vi "GEOM_findAmplifierbyCoord.vi"(9 "amplifiers":T1[](array[typedef]) {"fliped" items=["none", "horizontal", "vertical"]; "type" items=["LL", "LR", "UL", "UR"]}, 10 "ycoord":i32, 11 "xcoord":i32) -> (1 "amplifiers":T1[](array[typedef]) {"fliped" items=["none", "horizontal", "vertical"]; "type" items=["LL", "LR", "UL", "UR"]}, 2 "indexes":i32[](array[numeric]))   [LabVIEW 2016]
uses:
  GEOM_Amplifier.ctl
  GEOM_AmpType.ctl
  GEOM_ROI.ctl
  GEOM_Coords.ctl
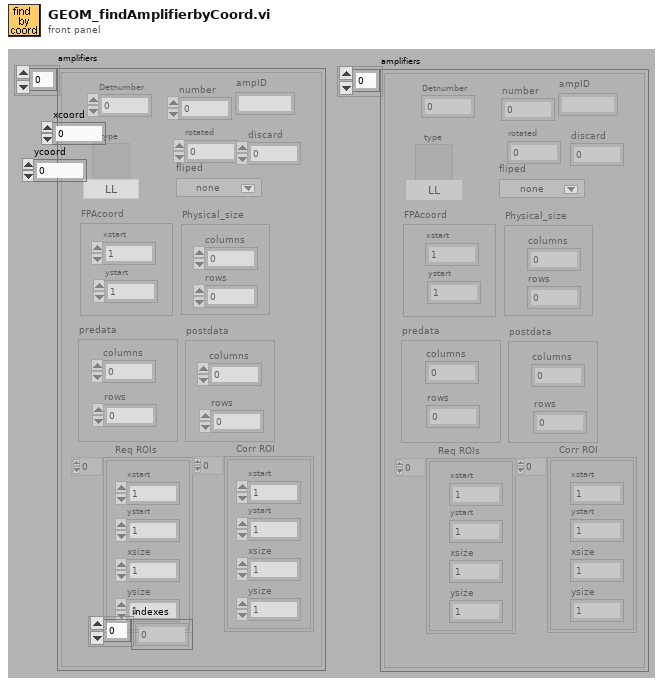
[diagram p1: front panel]
types:
  T1 = typedef "GEOM_Amplifier.ctl" = cluster{"number":i32, "type":T2, "rotated":i16, "fliped":u16, "FPAcoord":cluster{"xstart":i32, "ystart":i32}, "Physical_size":cluster{"columns":i32, "rows":i32}, "predata":cluster{"columns":i32, "rows":i32}, "postdata":cluster{"columns":i32, "rows":i32}, "Req ROIs":T3, "Corr ROI":T3, "Detnumber":i32, "ampID":string, "discard":i32}
  T2 = typedef "GEOM_AmpType.ctl" = u16
  T3 = typedef "GEOM_ROI.ctl" = T4[]
  T4 = typedef "GEOM_Coords.ctl" = cluster{"xstart":u32, "ystart":u32, "xsize":u32, "ysize":u32}
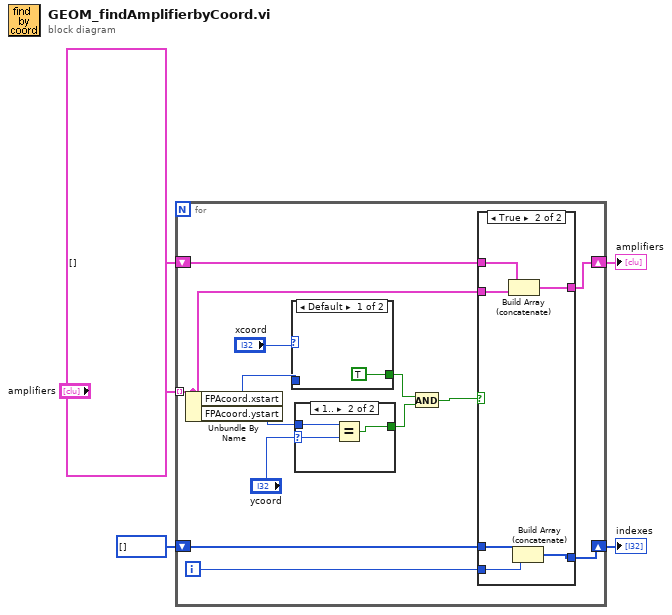
[diagram p0: block diagram]
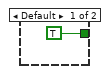
[diagram p3: hidden frame]
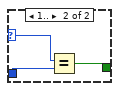
[diagram p4: hidden frame]
diagram:
  n1 = for {
    tunnel: "amplifiers" -> [w11] mode=indexing
    shift-right: [w10] -> w4
    shift-left: T1[] [] -> [w9]
    shift-right: [w7] -> w3
    shift-left: i32[] [] -> [w6]
    i -> [w8]
    n2 = Unbundle By Name(w11) -> ("FPAcoord.xstart"=w18:i32, "FPAcoord.ystart"=w17:i32)
    n3 = case shown="Default" "xcoord" {
      selector: "xcoord" -> [_ w32]
      tunnel: w18 -> [_ w34]
      tunnel: [TRUE w33] -> w16
      frame Default {
      }
      frame 1.. {
        n4 = Equal?(x=w32, y=w34) -> (x = y?=w33:bool)
      }
    }
    n5 = case shown="1.." "ycoord" {
      selector: "ycoord" -> [_ w28]
      tunnel: w17 -> [_ w30]
      tunnel: [TRUE w29] -> w15
      frame Default {
      }
      frame 1.. {
        n6 = Equal?(x=w30, y=w28) -> (x = y?=w29:bool)
      }
    }
    n7 = And(x=w16, y=w15) -> (x .and. y?=w12:bool)
    n8 = case shown="True" w12 {
      tunnel: w11 -> [_ w26]
      tunnel: [w20 w25] -> w10
      tunnel: w9 -> [w20 w24]
      tunnel: w8 -> [_ w22]
      tunnel: [w19 w21] -> w7
      tunnel: w6 -> [w19 w23]
      frame False {
      }
      frame True {
        n9 = Build Array (concatenate)(w24, w26) -> (w25:T1[])
        n10 = Build Array (concatenate)(w23, w22) -> (w21:i32[])
      }
    }
  }
  "amplifiers" <- w4
  "indexes" <- w3
